vi "process.vi"(8 "error in (no error)":errorcluster, 10 "Path":path=path "C:/LSST_TS/SystemSW/ts_sallabviewrt_tools/ts_sallv_exa/VIs/EXA_Connect.vi", 11 "VI in":refnum<class "VI.lvclass">) -> (0 "error out":errorcluster, 3 "VI out":refnum<class "VI.lvclass">)   [LabVIEW 2016, in "VI.lvclass"]
uses:
  VI.lvclass
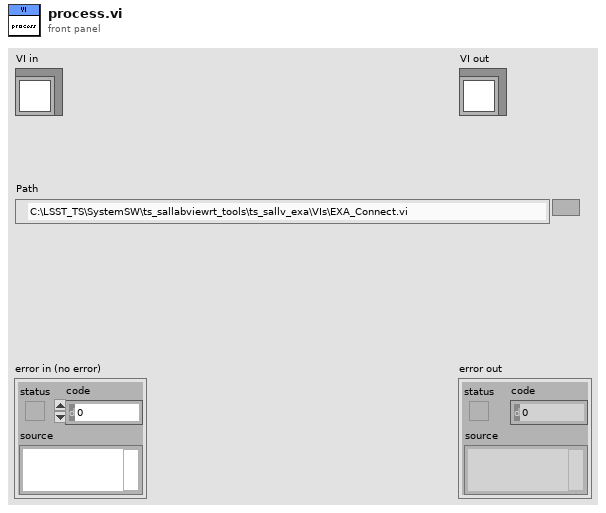
[diagram p1: front panel]
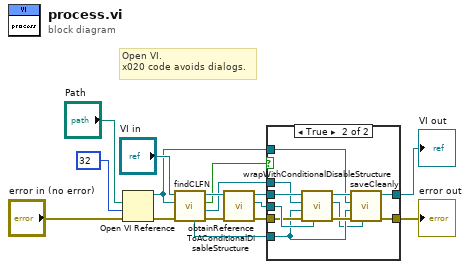
[diagram p0: block diagram]
diagram:
  # "Open VI.\nx020 code avoids dialogs."
  n1 = Open VI Reference(vi path="Path", options=32, error in (no error)="error in (no error)") -> (vi reference=w1:refnum<vi>, error out=w14:errorcluster)  [unwired: 3 in]
  n2 = call "findCLFN.vi"("error in (no error)"=w14, "vi reference"=w1, "VI in"="VI in") -> ("error out"=w5:errorcluster, "Node Refnum CLFN"=w9:refnum<vi>, "found?"=w11:bool, "VI out"=w12:refnum<class "VI.lvclass">, "Block Diagram"=w8:refnum<vi>)  [unwired: 4 in]
  n3 = call "obtainReferenceToAConditionalDisableStructure.vi"("error in (no error)"=w5, "VI in"=w12) -> ("error out"=w4:errorcluster, "Node Refnum CDS Source"=w7:refnum<vi>, "VI out"=w10:refnum<class "VI.lvclass">)  [unwired: 7 in]
  n4 = case shown="True" w11 {
    tunnel: w10 -> [w17 w29]
    tunnel: w9 -> [_ w28]
    tunnel: w8 -> [_ w21]
    tunnel: w7 -> [_ w27]
    tunnel: w4 -> [w18 w25]
    tunnel: [w18 w23] -> w3
    tunnel: [w17 w20] -> w2
    tunnel: w1 -> [_ w22]
    frame False {
    }
    frame True {
      n5 = call "wrapWithConditionalDisableStructure.vi"("Node Refnum CDS Source"=w27, "error in (no error)"=w25, "Block Diagram"=w21, "Node Refnum CLFN"=w28, "VI in"=w29) -> ("error out"=w24:errorcluster, "Node Refnum CDS New"=w19:refnum<vi>, "VI out"=w26:refnum<class "VI.lvclass">)  [unwired: 4 in]
      n6 = call "saveCleanly.vi"("Node Refnum CDS New"=w19, "error in (no error)"=w24, "Block Diagram"=w21, "vi reference"=w22, "VI in"=w26) -> ("error out"=w23:errorcluster, "VI out"=w20:refnum<class "VI.lvclass">)  [unwired: 5 in]
    }
  }
  "error out" <- w3
  "VI out" <- w2
